vi "GetSaveFilepath.vi"(8 "error in (no error)":errorcluster, 11 "UI_Interaction_Manager in":refnum<class "UI_Interaction_Manager.lvclass">) -> (0 "error out":errorcluster, 1 "OK?":bool, 2 "Selected Filepath":path, 3 "UI_Interaction_Manager out":refnum<class "UI_Interaction_Manager.lvclass">)   [LabVIEW 2011, in "UI_Interaction_Manager.lvclass"]
uses:
  UI_Interaction_Manager.lvclass
  UI_Interaction_Manager.lvclass/UI_Interaction_Manager.ctl
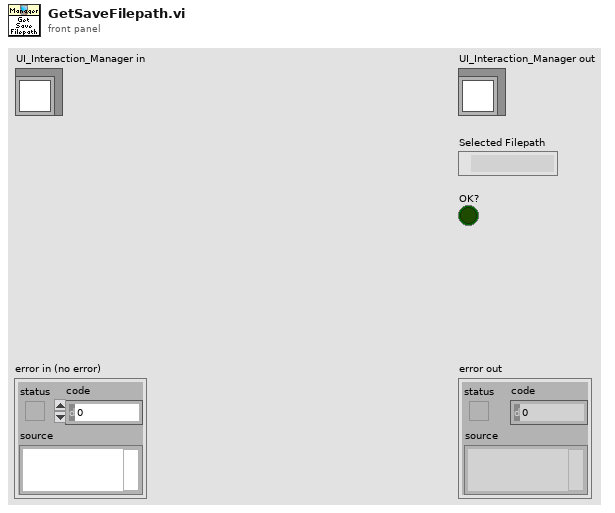
[diagram p1: front panel]
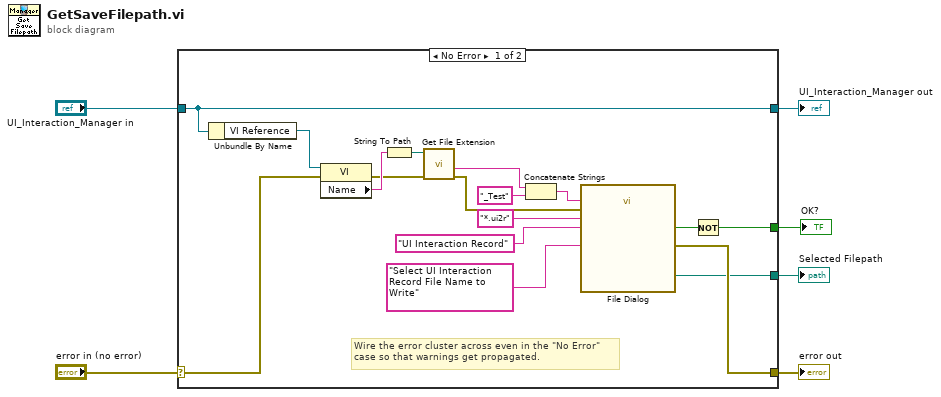
[diagram p0: block diagram]
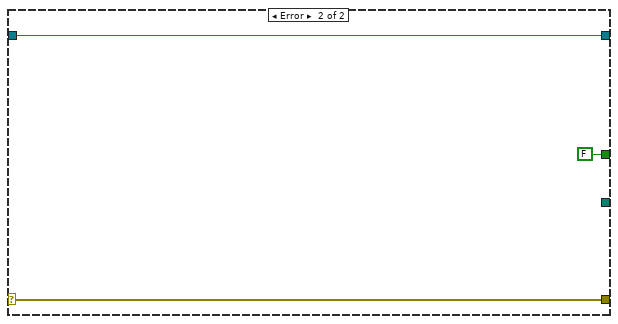
[diagram p2: hidden frame]
diagram:
  n1 = case shown="No Error" "error in (no error)" {
    selector: "error in (no error)" -> [w18 w26]
    tunnel: [w15 w26] -> w5
    tunnel: [w20 w25] -> w3
    tunnel: "UI_Interaction_Manager in" -> [w20 w25]
    tunnel: [w12 FALSE ("cancelled")] -> w2
    tunnel: [w14 _] -> w1
    frame No Error {
      # "Wire the error cluster across even in the \"No Error\"\ncase so that warnings get propagated."
      n2 = Unbundle By Name(w20) -> ("VI Reference"=w19:refnum<vi>)
      n3 = property class="VI"(reference=w19, error in=w18) -> (error out=w9:errorcluster, "Name"=w10:string)  [unwired: 1 out]
      n4 = String To Path(string=w10) -> (path=w11:path)
      n5 = call <vilib>:"Get File Extension.vi"("error in (no error)"=w9, "file"=w11) -> ("error out"=w8:errorcluster, "filename without extension"=w7:string)  [unwired: 6 in, 2 out]
      n6 = Concatenate Strings(w7, "_Test" ("string")) -> (w16:string)
      n7 = call "File Dialog"("prompt"="Select UI Interaction Record File Name to Write", "default name"=w16, "error in"=w8, "pattern (all files)"="*.ui2r", "pattern label"="UI Interaction Record") -> ("selected path"=w14:path, "cancelled"=w13:bool, "error out"=w15:errorcluster)  [unwired: 7 in, 1 out]
      n8 = Not(x=w13) -> (.not. x?=w12:bool)
    }
    frame Error {
    }
  }
  "error out" <- w5
  "UI_Interaction_Manager out" <- w3
  "OK?" <- w2
  "Selected Filepath" <- w1
